vi "TapeTeleOp.vi"(9 "Axes":dbl[](array[numeric]), 10 "Buttons":bool[](array[boolean]), 11 "Robot":T1) -> ()   [LabVIEW 2015]
uses:
  Robot Type Def.ctl
  Framework/JoystickMappingNamesTypeDef.ctl
  Lift/TW Global.vi
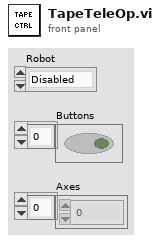
[diagram p1: front panel]
types:
  T1 = typedef "Robot Type Def.ctl" = enum32{"Disabled", "Ghost", "Casper", "Lofty", "Board", "RaceRobot", "Casper 2.0", "Excalibot 2.0"}
  T2 = typedef "JoystickMappingNamesTypeDef.ctl" = enum16{"Shoot Button", "Retrieve Button", "Arm Control", "High Gear", "Low Gear", "Enable PTO", "Disable PTO", "PortC Control", "PortC Up", "PortC Down", "Lift Control", "Drive VBus", "Override Arm Limits"}
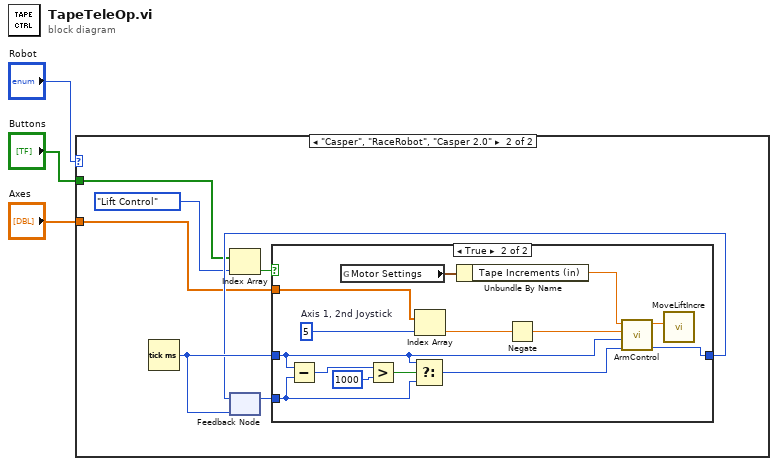
[diagram p0: block diagram]
diagram:
  n1 = case shown="\"Casper\", \"RaceRobot\", \"Casper 2.0\"" "Robot" {
    tunnel: "Axes" -> [_ w5]
    tunnel: "Buttons" -> [_ w4]
    frame "Disabled", Default {
    }
    frame "Casper", "RaceRobot", "Casper 2.0" {
      n2 = Tick Count (ms)() -> (millisecond timer value=w10:u32)
      n3 = Index Array(array=w4, index=JoystickMappingNamesTypeDef."Lift Control" ("Joystick Button Names")) -> (element=w7:bool)
      n4 = feedback #1(w10) -> (w9:u32)
      n5 = case shown="True" w7 {
        tunnel: [w11 w20] -> w8
        tunnel: w9 -> [_ w18]
        tunnel: w10 -> [w11 w19]
        tunnel: w5 -> [_ w17]
        frame False {
        }
        frame True {
          w25 = 5  # Axis 1, 2nd Joystick
          n6 = Subtract(x=w19, y=w18) -> (x-y=w24:u32)
          n7 = global read "TW Global.vi" "Motor Settings"() -> (w15:cluster{"Tape Increments (in)":dbl})
          n8 = Greater?(x=w24, y=u32 1000) -> (0:w22:bool)
          n9 = Select(t=w19, s=w22, f=w18) -> (s? t:f=w21:u32)
          n10 = Index Array(array=w17, index=w25) -> (element=w13:dbl)
          n11 = Unbundle By Name(w15) -> ("Tape Increments (in)"=w14:dbl)
          n12 = Negate(x=w13) -> (-x=w12:dbl)
          n13 = call "ArmControl.vi"("Last Increment time"=w21, "Current time"=w19, "Joystick"=w12, "Increment"=w14) -> ("Last Time"=w20:u32, "Increment Amount"=w16:dbl)  [unwired: 6 in]
          n14 = call "MoveLiftIncre.vi"("Distance (in)"=w16) -> ()  [unwired: 10 in, 1 out]
        }
      }
      n15 = feedback-in #1(w8) -> ()
    }
  }
